vi "find device.vi"(8 "error in (no error)":errorcluster, 11 "USB IO in":refnum<class "USB IO.lvclass">) -> (0 "error out":errorcluster, 3 "USB IO out":refnum<class "USB IO.lvclass">)   [LabVIEW 2025, in "USB IO.lvlib" / "USB IO.lvclass"]
uses:
  USB IO.lvclass
  USB IO.lvclass/USB IO.ctl
  <resource>/objmgr/daqmx.rc
panel:
  out "DO.Ports":tag[](array[tag])
  out "DO.Lines":tag[](array[tag])
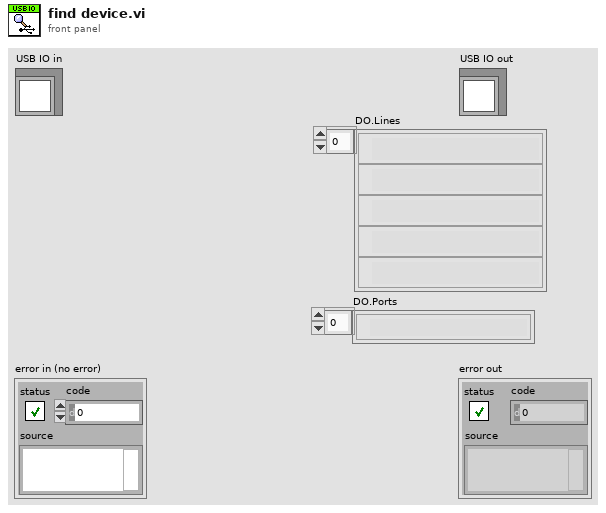
[diagram p1: front panel]
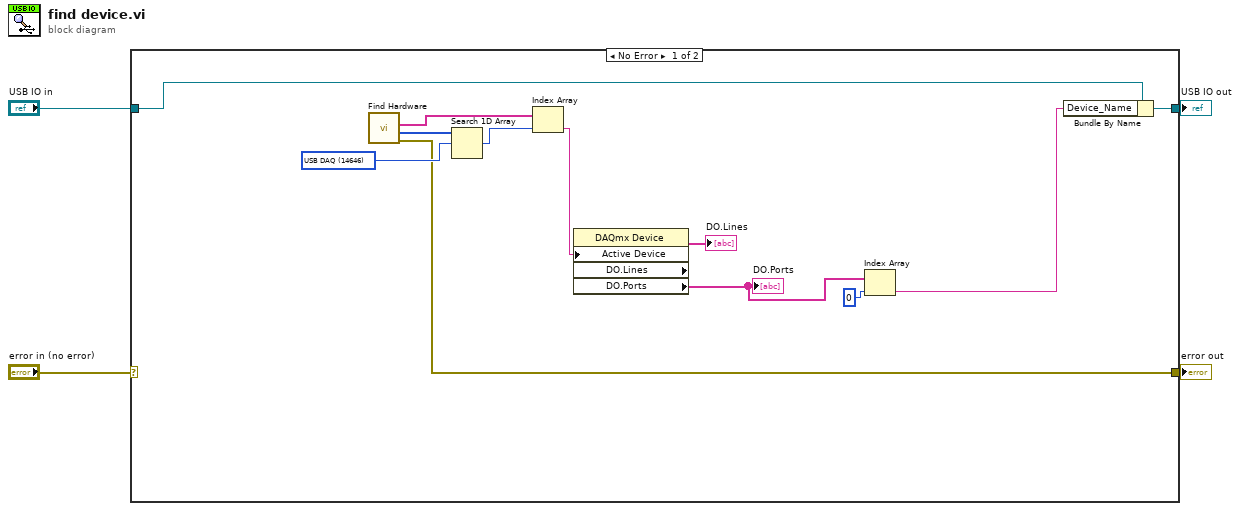
[diagram p0: block diagram]
diagram:
  n1 = case shown="No Error" "error in (no error)" {
    selector: "error in (no error)" -> [_ w18]
    tunnel: [w10 w18] -> w3
    tunnel: [w12 w17] -> w1
    tunnel: "USB IO in" -> [w11 w17]
    frame No Error {
      w15 = 14646 items=["M Series DAQ"=14643, "X Series DAQ"=15858, "E Series DAQ"=14642, "S Series DAQ"=14644, "B Series DAQ"=14662, "SC Series DAQ"=14645, "USB DAQ"=14646, "AO Series"=14647, "Digital I/O"=14648, "TIO Series"=14661, "Dynamic Signal Acquisition"=14649, "Switches"=14650, "CompactDAQ Chassis"=14658, "CompactRIO Chassis"=16144, "C Series Module"=14659, "SCXI Module"=14660, "SCC Connector Block"=14704, "SCC Module"=14705, "NI ELVIS"=14755, "Network DAQ"=14829, "SC Express"=15886, "FieldDAQ"=16151, "TestScale Chassis"=16180, "TestScale Module"=16181, "mioDAQ"=16182, "Unknown"=12588] ("ProductCategory")
      n2 = call "Find Hardware.vi"() -> ("error out"=w10:errorcluster, "Product Category"=w16:i32[], "DevNames"=w14:tag[])  [unwired: 8 in, 1 out]
      n3 = Search 1D Array(1D array=w16, element=w15) -> (index of element=w13:i32)  [unwired: 1 in]
      n4 = Index Array(array=w14, index=w13) -> (element=w9:tag)
      n5 = property class="DAQmx Device"("Active Device"=w9) -> ("DO.Lines"=→"DO.Lines":tag[], "DO.Ports"=w7:tag[])  [unwired: 2 in, 2 out]
      "DO.Ports" <- w7
      n6 = Index Array(array=w7, index=0) -> (element=w5:tag)
      n7 = Bundle By Name(cluster=w11, "Device_Name"=w5) -> (w12:refnum<class "USB IO.lvclass">)
    }
    frame Error {
    }
  }
  "error out" <- w3
  "USB IO out" <- w1
